vi "WSVCAP SHL FPGA LL SPI Build Write Memory Address.vi"(10 "Write CMD [1-4]":u8, 11 "Write Bit Index [0-39]":u8) -> (3 "Memory Address":u32)   [LabVIEW 2012]
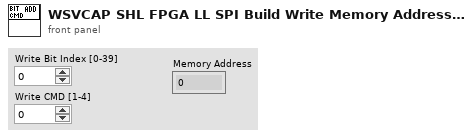
[diagram p1: front panel]
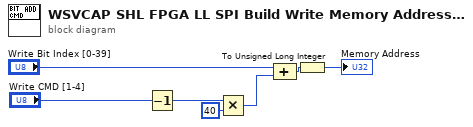
[diagram p0: block diagram]
diagram:
  n1 = Decrement(x="Write CMD [1-4]") -> (x-1=w7:u8)
  n2 = Multiply(x=w7, y=u8 40) -> (x*y=w5:u8)
  n3 = Compound Arithmetic op=ADD("Write Bit Index [0-39]", w5) -> (w4:u8)
  n4 = To Unsigned Long Integer(number=w4) -> (unsigned 32bit integer=→"Memory Address":u32)
